vi "Flappy Practice.vi"() -> ()   [LabVIEW 2017, in "Flappy Bird.lvlib"]
uses:
  Flappy Bird.lvlib
panel:
  out "current score":sgl
  in  "Quit":bool
  in  "Start":bool
  in  "Flap Button":bool
  out "XY Graph":cluster{"x":sgl[], "y_upper":dbl[]}[](graph)
  in  "Difficulty":dbl(knob) min=0.0 max=2.0 step=1.0 scale=0.0..2.0 scale format="%1d"
  in  "error in":errorcluster
  out "error out":errorcluster
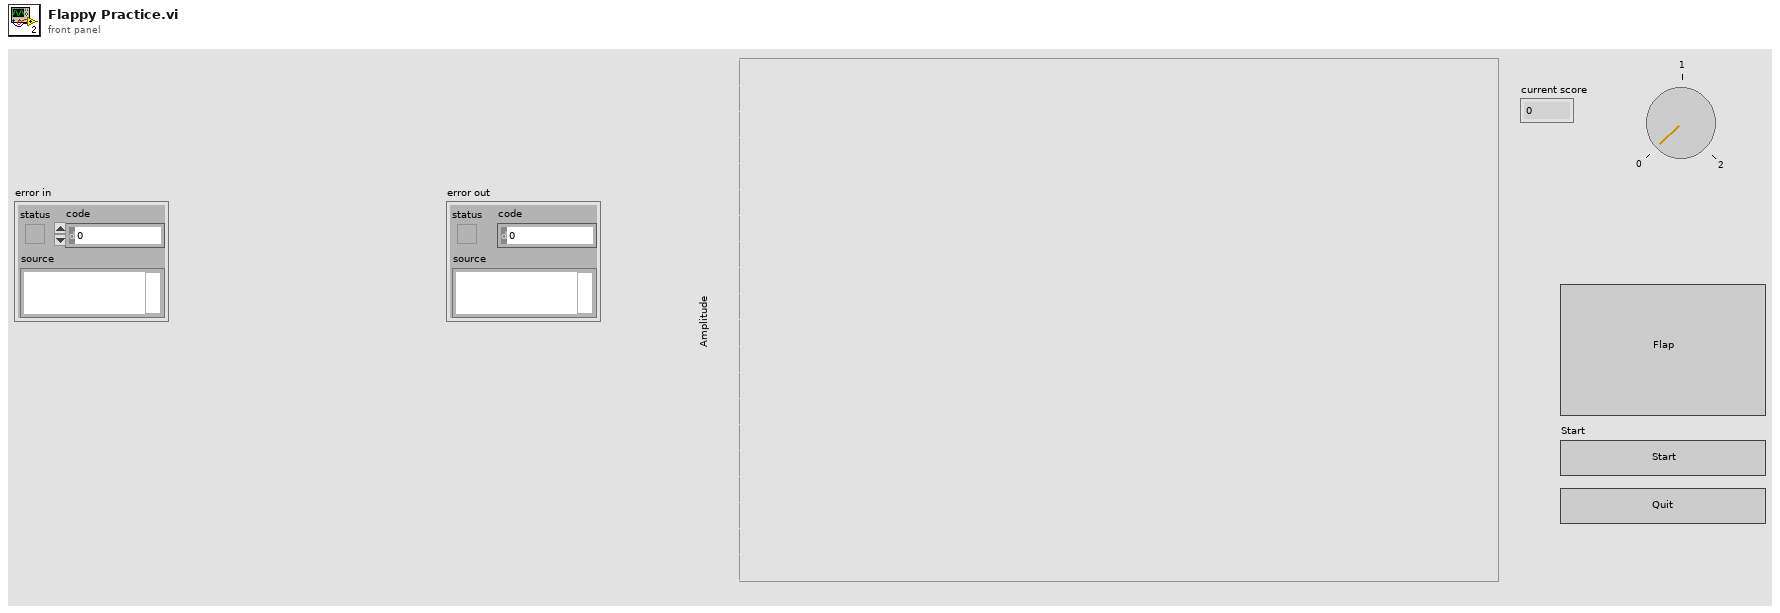
[diagram p1: front panel]
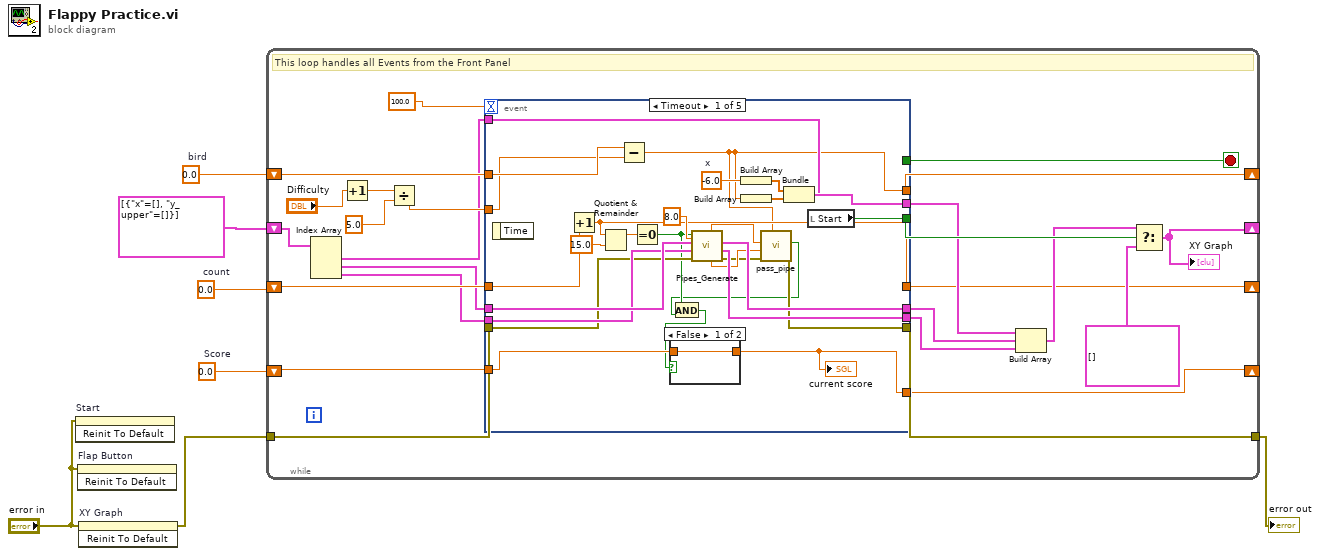
[diagram p0: block diagram]
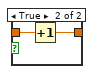
[diagram p2: hidden frame]
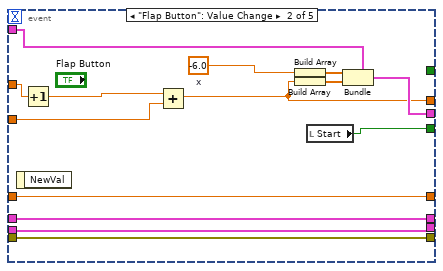
[diagram p3: hidden frame]
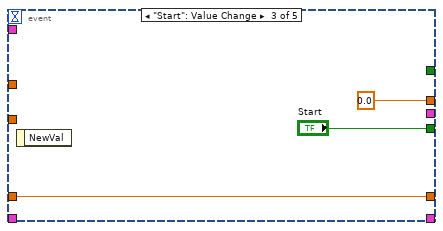
[diagram p4: hidden frame]
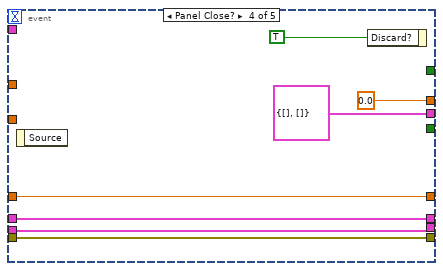
[diagram p5: hidden frame]
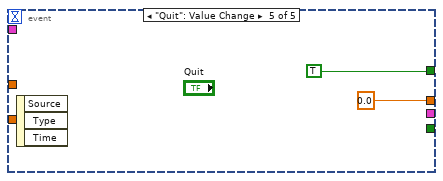
[diagram p6: hidden frame]
diagram:
  w1 = 0.0  # Score
  w4 = 0.0  # count
  w7 = 0.0  # bird
  n1 = invoke on="Start" class="Bool (strict)" method="Reinit To Default"(error in="error in") -> ()  [unwired: 2 in, 3 out]
  n2 = invoke on="Flap Button" class="Bool (strict)" method="Reinit To Default"(error in="error in") -> ()  [unwired: 2 in, 3 out]
  n3 = invoke on="XY Graph" class="XYGraph (strict)" method="Reinit To Default"(error in="error in") -> (error out=w6:errorcluster)  [unwired: 2 in, 2 out]
  n4 = while {
    shift-right: [w29] -> _
    shift-left: w7 -> [w28]
    tunnel: w6 -> [w12]
    tunnel: [w11] -> w5
    shift-right: [w13] -> _
    shift-left: w4 -> [w20]
    shift-right: [w14] -> _
    shift-left: cluster{"x":sgl[], "y_upper":dbl[]}[] [{"x"=[], "y_upper"=[]}] -> [w18]
    shift-right: [w8] -> _
    shift-left: w1 -> [w9]
    stop <- w32 stop-if-true
    # "This loop handles all Events from the Front Panel"
    n5 = Index Array(array=w18) -> (element #1=w17:cluster{"x":sgl[], "y_upper":dbl[]}, element #2=w16:cluster{"x":sgl[], "y_upper":dbl[]}, element #3=w15:cluster{"x":sgl[], "y_upper":dbl[]})  [unwired: 3 in]
    n6 = Increment(x="Difficulty") -> (x+1=w25:dbl)
    n7 = Divide(x=w25, y=5.0 ("x")) -> (x/y=w27:dbl)
    n8 = event shown="[0] Timeout" {
      selector: _ -> [_ _ _ _ _]
      dyn-events: _ -> [_ _ _ _ _]
      timeout: 100.0 ("x") -> [_ _ _ _ _]
      tunnel: [_ _ _ _ TRUE] -> w32
      tunnel: [w55 w72 _ cluster{sgl[], sgl[]} {[], []} _] -> w24
      tunnel: w28 -> [w56 w77 _ _ _]
      tunnel: [w57 w69 "Start" _ _] -> w30
      tunnel: [w42 w65 sgl 0.0 sgl 0.0 sgl 0.0] -> w29
      tunnel: w27 -> [w51 w64 _ _ _]
      tunnel: [w54 w68 _ w82 _] -> w22
      tunnel: [w53 w66 _ w83 _] -> w21
      tunnel: w20 -> [w52 w70 w78 w84 _]
      tunnel: w17 -> [w49 w71 _ _ _]
      tunnel: w16 -> [w48 w66 _ w83 _]
      tunnel: w15 -> [w47 w68 _ w82 _]
      tunnel: [w45 w70 w78 w84 _] -> w13
      tunnel: w12 -> [w46 w67 _ w81 _]
      tunnel: [w38 w67 _ w81 _] -> w11
      tunnel: w9 -> [w36 _ _ _ _]
      tunnel: [w35 _ _ _ _] -> w8
      event Timeout {
        w60 = sgl -6.0  # x
        n9 = event-data() -> ()  [unwired: 1 in, 1 out]
        n10 = Increment(x=w52) -> (x+1=w45:dbl)
        n11 = Quotient & Remainder(x=w45, y=15.0) -> (x-y*floor(x/y)=w43:dbl)  [unwired: 1 out]
        n12 = Subtract(x=w56, y=w51) -> (x-y=w42:dbl)
        n13 = Equal To 0?(x=w43) -> (x = 0?=w37:bool)
        n14 = call "Pipes_Generate.vi"("Opening Width"=8.0, "error in (no error)"=w46, "X&Y-Lower Lim"=w47, "X&Y-Upper Lim"=w48, "Gen Pipe"=w37) -> ("error out"=w39:errorcluster, "X&YUpper"=w54:cluster{"x":sgl[], "y_upper":sgl[]}, "X&YLower"=w53:cluster{"x":sgl[], "y_lower":sgl[]}, "Lower Limit"=w40:dbl, "Upper Limit"=w41:dbl)  [unwired: 2 in]
        n15 = Build Array(w60) -> (w59:sgl[])
        n16 = Build Array(w42) -> (w58:dbl[])
        n17 = call "pass_pipe.vi"("bird"=w42, "error in (no error)"=w39, "y lower"=w40, "y upper"=w41) -> ("error out"=w38:errorcluster, "pass"=w34:bool)  [unwired: 6 in]
        n18 = And(x=w37, y=w34) -> (x .and. y?=w33:bool)
        n19 = case shown="False" w33 {
          tunnel: w36 -> [w61 w63]
          tunnel: [w61 w62] -> w35
          frame False {
          }
          frame True {
            n20 = Increment(x=w63) -> (x+1=w62:dbl)
          }
        }
        "current score" <- w35
        n21 = Bundle(cluster=w49, "x"=w59, "y_upper"=w58) -> (w55:cluster{"x":sgl[], "y_upper":dbl[]})
        n22 = local read "Start"() -> (w57:bool)
      }
      event "Flap Button": Value Change {
        w76 = sgl -6.0  # x
        n23 = event-data() -> ()  [unwired: 1 in, 1 out]
        n24 = Increment(x=w77) -> (x+1=w73:dbl)
        n25 = Add(x=w73, y=w64) -> (x+y=w65:dbl)
        n26 = Build Array(w76) -> (w75:sgl[])
        n27 = Build Array(w65) -> (w74:dbl[])
        n28 = local read "Start"() -> (w69:bool)
        n29 = Bundle(cluster=w71, "x"=w75, "y_upper"=w74) -> (w72:cluster{"x":sgl[], "y_upper":dbl[]})
      }
      event "Start": Value Change {
        n30 = event-data() -> ()  [unwired: 1 in, 1 out]
      }
      event Panel Close? {
        n31 = event-data() -> ()  [unwired: 1 in, 1 out]
        n32 = event-data("Discard?"=TRUE) -> ()  [unwired: 1 in, 1 out]
      }
      event "Quit": Value Change {
        n33 = event-data() -> ()  [unwired: 1 in, 3 out]
      }
    }
    n34 = Build Array(w24, w21, w22) -> (w19:cluster{"x":sgl[], "y_upper":dbl[]}[])
    n35 = Select(t=w19, s=w30, f=cluster{"x":sgl[], "y_upper":dbl[]}[] [] ("appended array")) -> (s? t:f=w14:cluster{"x":sgl[], "y_upper":dbl[]}[])
    "XY Graph" <- w14
  }
  "error out" <- w5
